vi "SW Heartbeat Timer.vi"(8 "error in (no error)":errorcluster, 9 "Reset":bool, 10 "Pause":bool, 11 "Target Time":dbl format="%#_13g") -> (0 "error out":errorcluster, 2 "Time Elapsed":bool, 3 "Elapsed Time":dbl)   [LabVIEW 2017]
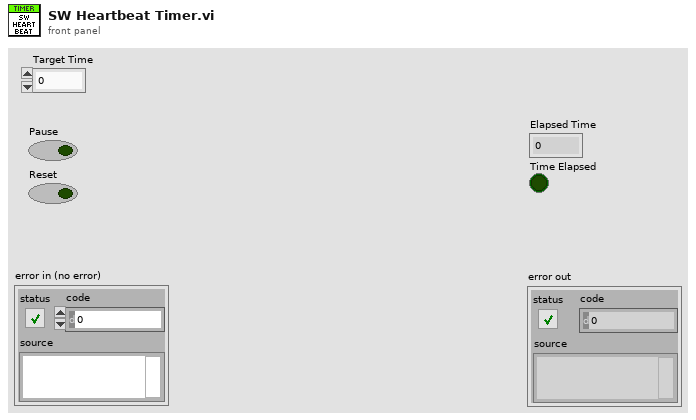
[diagram p1: front panel]
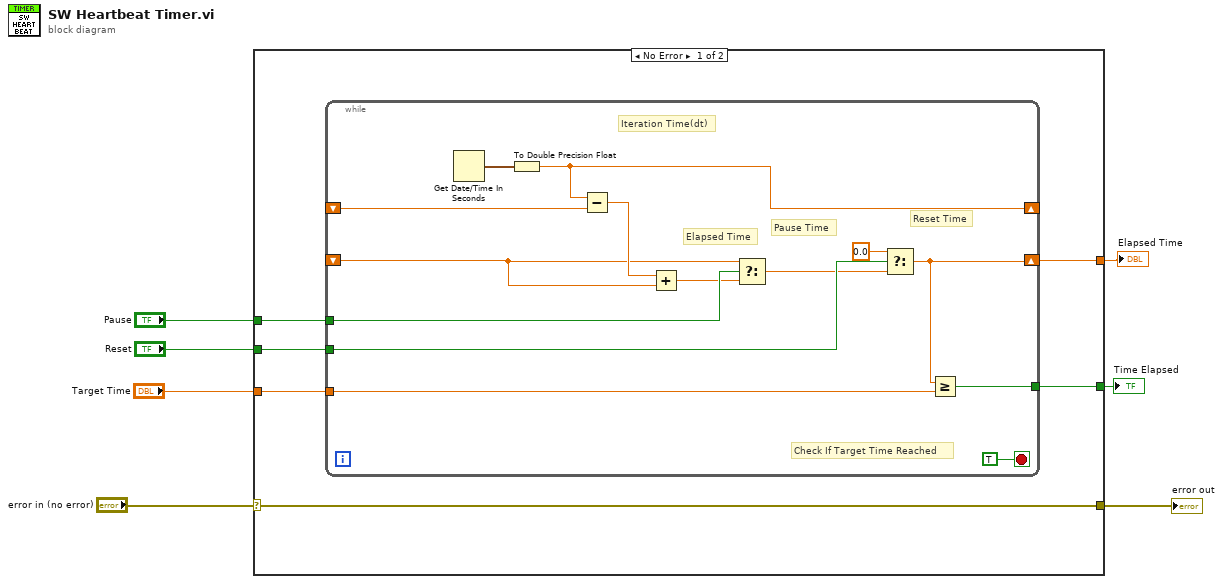
[diagram p0: block diagram]
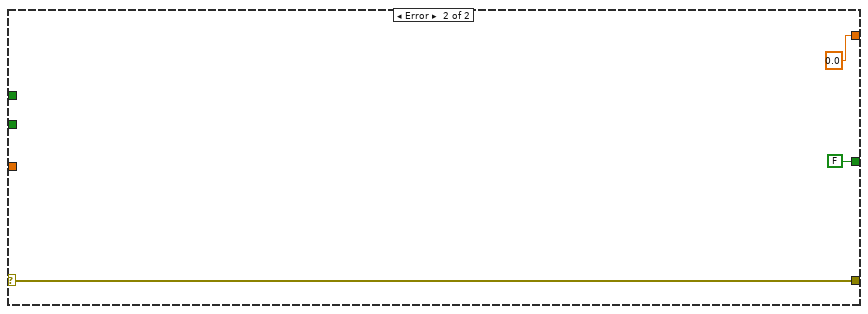
[diagram p2: hidden frame]
diagram:
  n1 = case shown="No Error" "error in (no error)" {
    selector: "error in (no error)" -> [w13 w30]
    tunnel: [w13 w30] -> w7
    tunnel: "Pause" -> [w12 _]
    tunnel: "Reset" -> [w11 _]
    tunnel: [w10 0.0 ("t")] -> w3
    tunnel: "Target Time" -> [w9 _]
    tunnel: [w8 FALSE] -> w1
    frame No Error {
      n2 = while {
        shift-right: [w25] -> _
        shift-left: _ -> [w24]
        shift-right: [w16] -> w10
        shift-left: _ -> [w20]
        tunnel: w12 -> [w22]
        tunnel: w11 -> [w19]
        tunnel: w9 -> [w15]
        tunnel: [w14] -> w8
        stop <- TRUE stop-if-true
        # "Check If Target Time Reached"
        # "Reset Time"
        # "Pause Time"
        # "Elapsed Time"
        # "Iteration Time(dt)"
        n3 = Get Date/Time In Seconds() -> (seconds since 1Jan1904=w26:timestamp)
        n4 = To Double Precision Float(number=w26) -> (double precision float=w25:dbl)
        n5 = Subtract(x=w25, y=w24) -> (x-y=w23:dbl)
        n6 = Add(x=w23, y=w20) -> (x+y=w21:dbl)
        n7 = Select(t=w20, s=w22, f=w21) -> (s? t:f=w17:dbl)
        n8 = Select(t=0.0, s=w19, f=w17) -> (s? t:f=w16:dbl)
        n9 = Greater Or Equal?(x=w16, y=w15) -> (x >= y?=w14:bool)
      }
    }
    frame Error {
    }
  }
  "error out" <- w7
  "Elapsed Time" <- w3
  "Time Elapsed" <- w1
